vi "0ZZTEMPZZ.vi"(0 "Time Target (s)":dbl=1.0, 2 "Reset":bool, 3 "Auto Reset":bool, 5 "error in (no error)":errorcluster, 8 "Set Start Time (s)":dbl) -> (11 "Get Start Time (s)":dbl, 13 "Start Time Text":string, 14 "Present (s)":dbl, 15 "Present Text":string, 16 "Elapsed Time (s)":dbl, 17 "Time has Elapsed":bool, 18 "Elapsed Time Text":string, 19 "error out":errorcluster)   [LabVIEW 2017]
doc: "Indicates the amount of time that has elapsed since the specified start time.\n--------------------\n\nThis Express VI is configured as follows:\n\nTime Target: 1 s\nAuto Reset: Off"
uses:
  Sense/Generate Instructions.vi
panel:
  # "Do a reset as soon as time has elapsed."
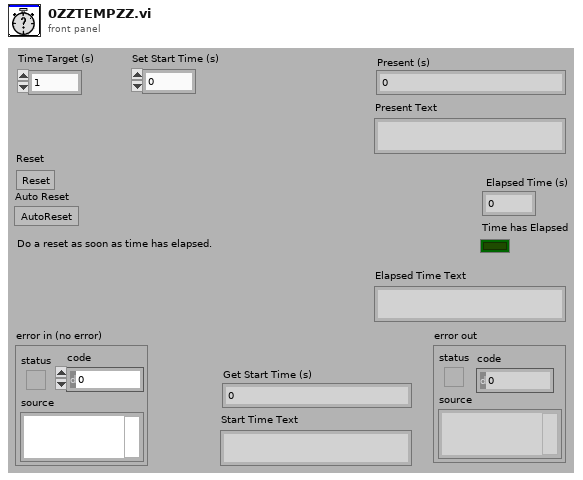
[diagram p1: front panel]
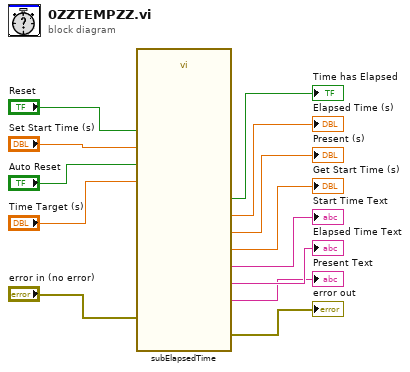
[diagram p0: block diagram]
diagram:
  n1 = call <vilib>:"subElapsedTime.vi"("Reset"="Reset", "Elapsed Time Target"="Time Target (s)", "Set Start Time"="Set Start Time (s)", "Auto Reset"="Auto Reset", "error in (no error)"="error in (no error)") -> ("Elapsed TimeText"=→"Elapsed Time Text":string, "Present Text"=→"Present Text":string, "Start Time Text"=→"Start Time Text":string, "Time has Elapsed"=→"Time has Elapsed":bool, "Elapsed Time"=→"Elapsed Time (s)":dbl, "Present"=→"Present (s)":dbl, "Get Start Time"=→"Get Start Time (s)":dbl, "error out"=→"error out":errorcluster)  [unwired: 7 in]
